vi "Receive.vi"(8 "错误输入（无错误）":errorcluster, 10 "CANChannel":u32, 11 "DeviceType":T2=3 items=["PCI-CAN200"=7, "USB-CAN"=2, "USB-CAN200"=3]) -> (0 "错误输出":errorcluster, 1 "VCI_CAN_OBJ_R":T1={"ID"=96, 0, 0, 0, "TimeStamp"=0, "TimeFlag"=0, "SendType"=0, "RemoteFlag"=0, "ExternFlag"=0, "DataLen"=8, "Byte0"=0, "Byte1"=248, "Byte2"=17, "Byte3"=0, "Byte4"=0, "Byte5"=0, "Byte6"=0, "Byte7"=0, "Channel"=0, 77, 32} {"Byte7" format="%x"; "Byte6" format="%x"; "Byte5" format="%x"; "Byte4" format="%x"; "Byte3" format="%x"; "Byte2" format="%x"; "Byte1" format="%x"; "Byte0" format="%x"}, 2 "Result":bool, 3 "DeviceTypeOut":u16(ring)=7 items=["PCI-CAN200"=7])   [LabVIEW 2013]
uses:
  DevType.ctl
  VCI_CAN.dll
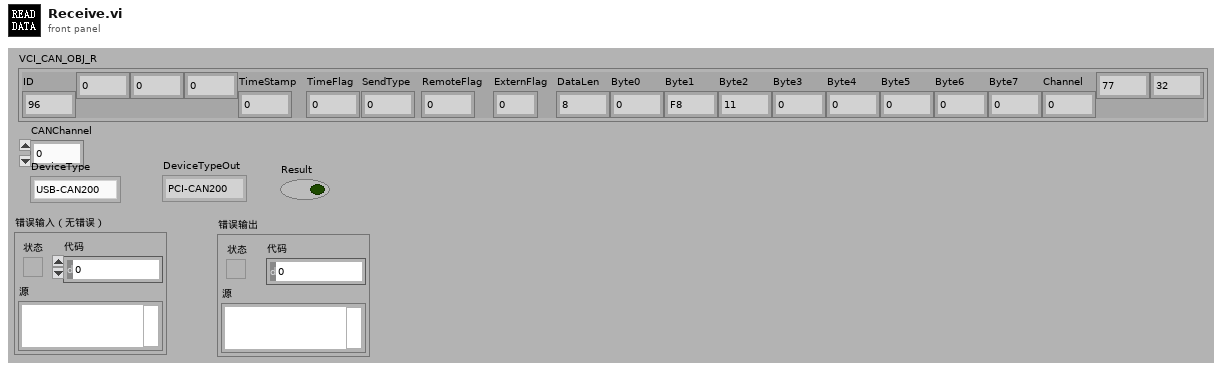
[diagram p1: front panel]
types:
  T1 = cluster{"ID":u8, u8, u8, u8, "TimeStamp":u32, "TimeFlag":u8, "SendType":u8, "RemoteFlag":u8, "ExternFlag":u8, "DataLen":u8, "Byte0":u8, "Byte1":u8, "Byte2":u8, "Byte3":u8, "Byte4":u8, "Byte5":u8, "Byte6":u8, "Byte7":u8, "Channel":u8, u8, u8}
  T2 = typedef "DevType.ctl" = u16
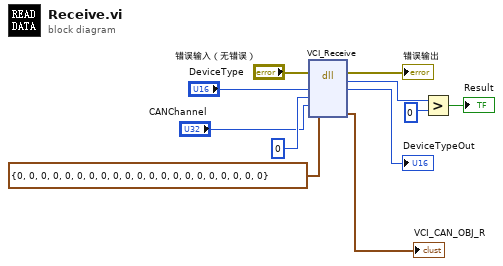
[diagram p0: block diagram]
diagram:
  n1 = dll-call lib="PTH1Mabs CUsers\nAdministratorDesktopCAN震动测试USB-CANVCI_CAN.dll" fn="VCI_Receive"(error in="错误输入（无错误）", "DeviceType"="DeviceType", "DeviceInd"=0, "CANInd"="CANChannel", "VCI_CAN_OBJ_R"=T1 {"ID"=0, 0, 0, 0, "TimeStamp"=0, "TimeFlag"=0, "SendType"=0, "RemoteFlag"=0, "ExternFlag"=0, "DataLen"=0, "Byte0"=0, "Byte1"=0, "Byte2"=0, "Byte3"=0, "Byte4"=0, "Byte5"=0, "Byte6"=0, "Byte7"=0, "Channel"=0, 0, 0} ("VCI_CAN_OBJ_R 2")) -> (error out=→"错误输出":errorcluster, "返回类型"=w7:u32, "DeviceType"=→"DeviceTypeOut":u32, "VCI_CAN_OBJ_R"=→"VCI_CAN_OBJ_R":T1)  [unwired: 4 in, 1 out]
  n2 = Greater?(x=w7, y=u32 0) -> (0:→"Result":bool)
